vi "ApplyLayoutToObject.vi"(5 "scaling settings":T1={"scaling factor"={"horizontal"=1.0, "vertical"=1.0}, "scaling to ignore"=variant} {"scaling factor"."vertical" min=0.0; "scaling factor"."horizontal" min=0.0}, 7 "properties to ignore":variant, 8 "error in (no error)":errorcluster, 10 "GObj Refnum":refnum<vi>, 11 "Cluster Control Layout in":refnum<class "Cluster Control Layout.lvclass">) -> (0 "error out":errorcluster, 3 "Cluster Control Layout out":refnum<class "Cluster Control Layout.lvclass">)   [LabVIEW 2010, in "NI_SE_Front Panel Layout.lvlib" / "Cluster Control Layout.lvclass"]
doc: "Apply layout information to the GObj Refnum."
uses:
  Cluster Control Layout.lvclass
  Scaling Factor_Options.ctl
  XY Scaling Factor.ctl
  Control Layout/Control Layout.lvclass
  Cluster Control Layout.lvclass/Cluster Control Layout.ctl
  Object Layout/Object Layout.lvclass/Object Layout.ctl
  Object Layout/Get UID.vi
  Object Layout/Get Unique Name.vi
  Convert UID To String.vi
  Properties To Ignore.vi
  NI_SE_Front Panel Layout.lvlib
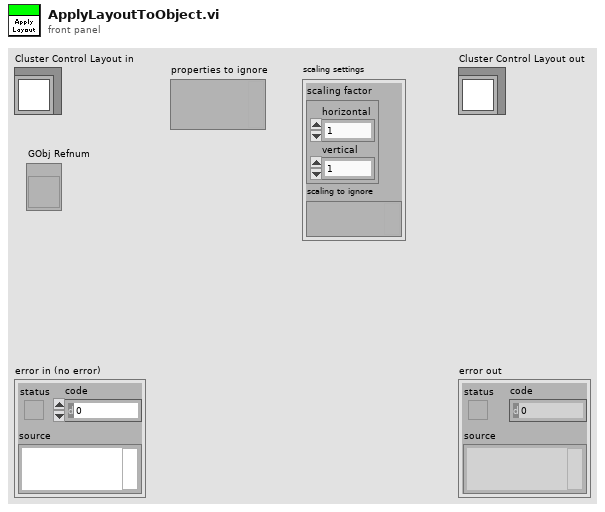
[diagram p1: front panel]
types:
  T1 = typedef "NI_SE_Front Panel Layout.lvlib/Scaling Factor_Options.ctl" = cluster{"scaling factor":T2, "scaling to ignore":variant}
  T2 = typedef "NI_SE_Front Panel Layout.lvlib/XY Scaling Factor.ctl" = cluster{"horizontal":dbl, "vertical":dbl}
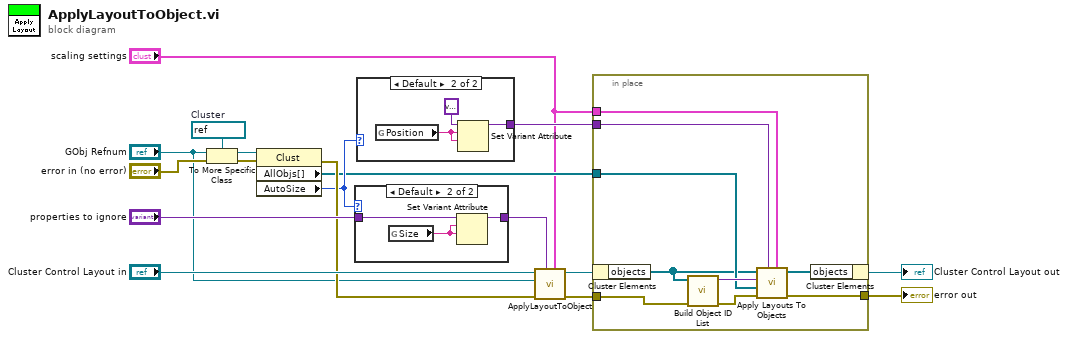
[diagram p0: block diagram]
diagram:
  w14 = refnum<vi> refnum  # Cluster
  n1 = To More Specific Class(target class=w14, reference="GObj Refnum", error in="error in (no error)") -> (specific class reference=w13:refnum<vi>, error out=w12:errorcluster)
  n2 = property class="Clust"(reference=w13, error in=w12) -> (error out=w10:errorcluster, "AllObjs[]"=w6:refnum<vi>[], "AutoSize"=w9:u32)  [unwired: 1 out]
  n3 = case shown="Default" w9 {
    tunnel: "properties to ignore" -> [w18 w21]
    tunnel: [w18 w20] -> w15
    frame 0 {
      # "0: no autosize"
    }
    frame Default {
      n4 = global read "Properties To Ignore.vi" "Size"() -> (w19:string)
      n5 = Set Variant Attribute(Variant=w21, name=w19, value=w19) -> (Variant out=w20:variant)  [unwired: 1 in, 2 out]
    }
  }
  n6 = case shown="Default" w9 {
    tunnel: [_ w23] -> w5
    frame 0, 1 {
      # "0: no autosize\n1: size to fit"
    }
    frame Default {
      n7 = global read "Properties To Ignore.vi" "Position"() -> (w22:string)
      n8 = Set Variant Attribute(Variant=variant ("variant"), name=w22, value=w22) -> (Variant out=w23:variant)  [unwired: 1 in, 2 out]
    }
  }
  n9 = call-parent "ApplyLayoutToObject.vi"("scaling settings"="scaling settings", "properties to ignore"=w15, "error in (no error)"=w10, "GObj Refnum"="GObj Refnum", "Control Layout in"="Cluster Control Layout in") -> ("error out"=w7:errorcluster, "Control Layout out"=w2:refnum<class "Cluster Control Layout.lvclass">)  [unwired: 5 in]
  n10 = in-place {
    in-place-border: w7 -> [w33]
    in-place-border: w6 -> [w31]
    in-place-border: w5 -> [w30]
    in-place-border: "scaling settings" -> [w29]
    in-place-border: [w27] -> w3
    n11 = in-place-cluster #1(w2) -> ("objects"=w26:refnum<class "Object Layout.lvclass">[])
    n12 = call "Build Object ID List.vi"("error in"=w33, "object layouts"=w26) -> ("error out"=w28:errorcluster, "object ID list"=w32:variant)  [unwired: 8 in]
    n13 = call "Apply Layouts To Objects.vi"("scaling settings"=w29, "properties to ignore"=w30, "error in"=w28, "GObj refnums"=w31, "object ID list in"=w32, "object layouts in"=w26) -> ("error out"=w27:errorcluster, "object layouts out"=w25:refnum<class "Object Layout.lvclass">[])  [unwired: 3 in, 1 out]
    n14 = in-place-cluster #1("objects"=w25) -> (→"Cluster Control Layout out":refnum<class "Cluster Control Layout.lvclass">)
  }
  "error out" <- w3
